vi "Append Character.vi"(9 "Character":string, 10 "String In":string) -> (2 "String Out":string)   [LabVIEW 2018, in "MVA Framework.lvlib" / "NumericKeypadDialogBox.lvlib" / "NumericKeypadDialogBox.lvclass"]
doc: "追加字符"
uses:
  NumericKeypadDialogBox.lvclass
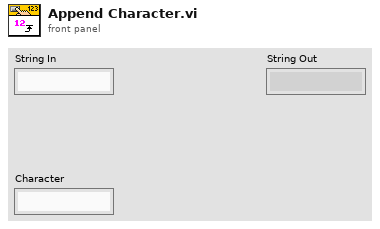
[diagram p1: front panel]
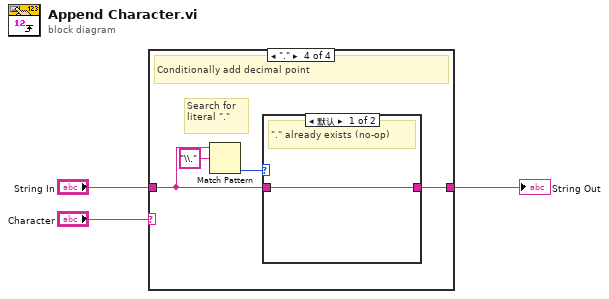
[diagram p0: block diagram]
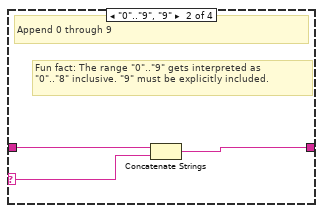
[diagram p3: hidden frame]
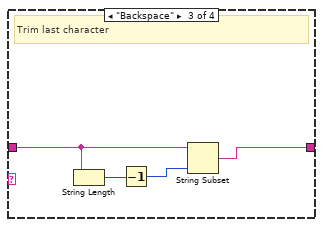
[diagram p4: hidden frame]
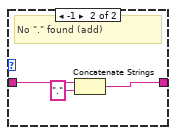
[diagram p5: hidden frame]
diagram:
  n1 = case shown="\".\"" "Character" {
    selector: "Character" -> [_ w5 _ _]
    tunnel: [w4 w7 w11 w12] -> w1
    tunnel: "String In" -> [w4 w6 w10 w13]
    frame Default {
      # "Unknown input"
    }
    frame "0".."9", "9" {
      # "Fun fact: The range \"0\"..\"9\" gets interpreted as\n\"0\"..\"8\" inclusive. \"9\" must be explicitly included."
      # "Append 0 through 9"
      n2 = Concatenate Strings(w6, w5) -> (w7:string)
    }
    frame "Backspace" {
      # "Trim last character"
      n3 = String Length(string=w10) -> (length=w9:i32)
      n4 = Decrement(x=w9) -> (x-1=w8:i32)
      n5 = String Subset(string=w10, length (rest)=w8) -> (substring=w11:string)  [unwired: 1 in]
    }
    frame "." {
      # "Search for\nliteral \".\""
      # "Conditionally add decimal point"
      n6 = Match Pattern(string=w13, regular expression="\\.") -> (offset past match=w14:i32)  [unwired: 1 in, 3 out]
      n7 = case shown="默认" w14 {
        tunnel: w13 -> [w16 w19]
        tunnel: [w16 w18] -> w12
        frame Default {
          # "\".\" already exists (no-op)"
        }
        frame -1 {
          # "No \".\" found (add)"
          n8 = Concatenate Strings(w19, "." ("string")) -> (w18:string)
        }
      }
    }
  }
  "String Out" <- w1
